vi "SCMain.vi"(0 "once?":bool, 1 "continousSequencer?":bool) -> ()   [LabVIEW 2014]
uses:
  <vilib>/Platform/TimedLoop/XDataNode/timing_clust.ctl
  <vilib>/Platform/TimedLoop/XDataNode/nitl_modes.ctl
  <vilib>/Platform/TimedLoop/XDataNode/wakeup.ctl
  SCGlobVars.vi
  <vilib>/rvi/Emulation/niFpgaSctlEmulationGetInTimedLoop.vi
  <vilib>/rvi/Emulation/niFpgaEmulationReportErrorSimple.vi
  <vilib>/rvi/Emulation/niFpgaGetClockAttributes.vi
  <vilib>/rvi/Emulation/niFpgaCriticalErrorInLSC.vi
  <vilib>/rvi/eio/common/nirviEmuTemplateMethod_errors.vi
  Sequencer/sequencerGlobVars.vi
  <vilib>/Platform/TimedLoop/XDataNode/XDataNode.xnode
  <vilib>/eio/EIONode/EIONode.xnode
  <vilib>/Platform/TimedLoop/XDataNode/XDNodeRunTimeDep.lvlib
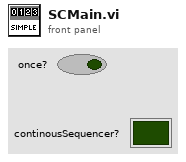
[diagram p1: front panel]
types:
  T1 = typedef "XDNodeRunTimeDep.lvlib/timing_clust.ctl" = cluster{"Expected End [f-1]":u64, "Actual End [f-1]":u64, "Finished Late? [f-1]":bool, "Expected End [i-1]":u64, "Actual End [i-1]":u64, "Finished Late? [i-1]":bool, "Expected Start [i]":u64, "Actual Start [i]":u64, "Expected Start [f]":u64, "Actual Start [f]":u64, "Source Name":string, "Structure Name":string, "Period":i64, "Deadline":i64, "Offset":i64, "Start":i64, "Priority":i32, "Timeout":i32, "Mode":T2, "Wakeup Reason":T3, "Error":errorcluster, "Source Type":string, "Secondary Source Type":string, "Global End Time":u64, "Global Start Time":u64, "Frame Duration":u64, "Iteration Duration":u64, "Assigned CPU":i32, "I/O Scan Engine Mode":u32}
  T2 = typedef "XDNodeRunTimeDep.lvlib/nitl_modes.ctl" = enum32{"No Change", "Process missed periods, maintain original phase", "Discard missed periods, maintain original phase", "Process missed periods, ignore original phase", "Discard missed periods, ignore original phase"}
  T3 = typedef "XDNodeRunTimeDep.lvlib/wakeup.ctl" = enum32{"Normal", "Aborted", "Asynchronous wakeup", "Timing source error", "Timed loop error", "Timeout"}
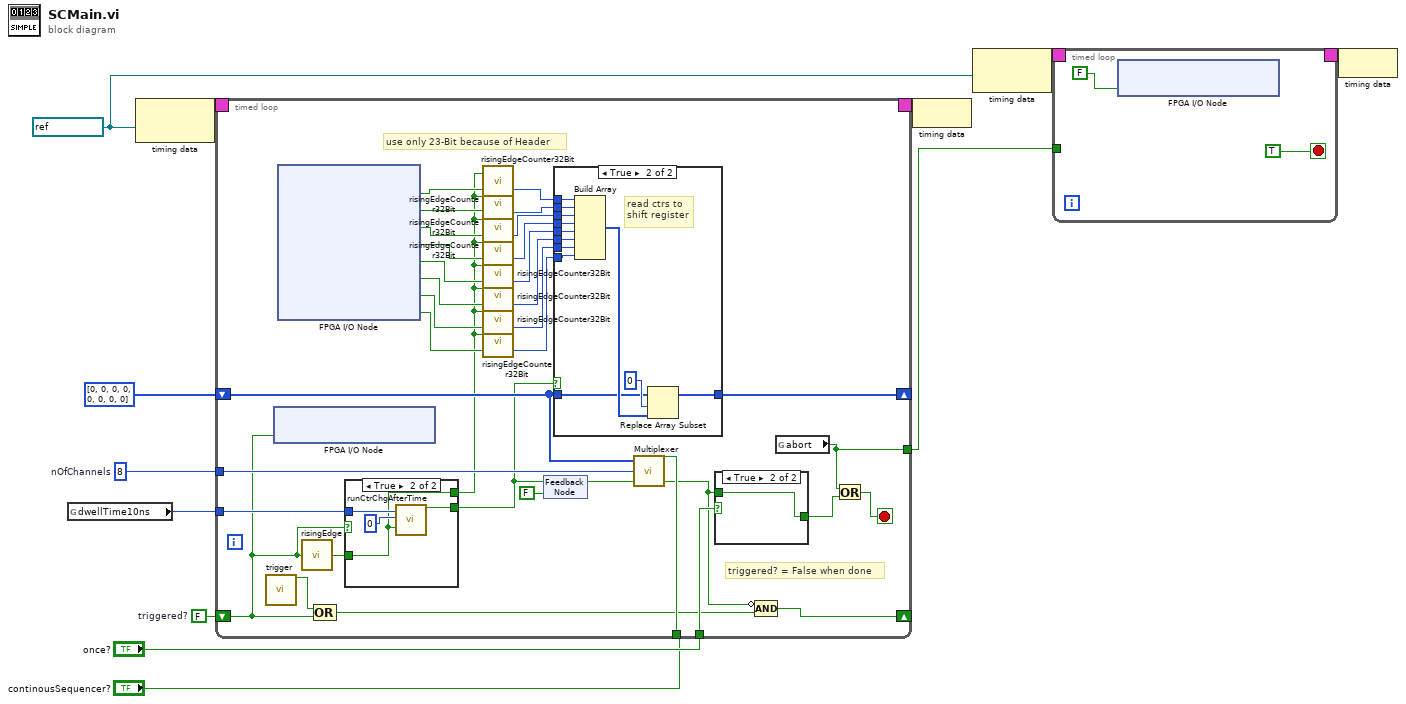
[diagram p0: block diagram]
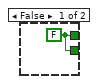
[diagram p2: hidden frame]
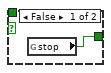
[diagram p3: hidden frame]
diagram:
  w1 = FALSE  # triggered?
  w9 = u8 8  # nOfChannels
  w3 = refnum<k21> "100MHz" ("Source Name")
  n1 = global read "SCGlobVars.vi" "dwellTime10ns"() -> (w5:u32)
  n2 = node-c288(w3) -> (w12:T1)
  n3 = timed-loop {
    timing: w12 -> [_]
    timing-out: [_] -> w11
    shift-right: [w31] -> _
    shift-left: u32[] [0, 0, 0, 0, 0, 0, 0, 0] -> [w28]
    tunnel: w9 -> [w26]
    tunnel: w5 -> [w30]
    tunnel: "once?" -> [w25]
    tunnel: "continousSequencer?" -> [w24]
    tunnel: [w21] -> w2
    shift-right: [w19] -> _
    shift-left: w1 -> [w13]
    stop <- w22 stop-if-true
    # "triggered? = False when done"
    # "use only 23-Bit because of Header"
    n4 = call "trigger.vi"() -> ("triggered"=w20:bool)  [unwired: 19 in]
    n5 = xnode "FPGA I/O Node"("SPScanFlagDio11Con1"=w13) -> ()  [unwired: 1 in, 1 out]
    n6 = xnode "FPGA I/O Node"() -> ("Connector1/DIO16"=w47:bool, "Connector1/DIO17"=w46:bool, "Connector1/DIO18"=w45:bool, "Connector1/DIO19"=w44:bool, "Connector1/DIO20"=w43:bool, "Connector1/DIO21"=w42:bool, "Connector1/DIO22"=w41:bool, "Connector1/DIO23"=w40:bool)  [unwired: 8 in, 8 out]
    n7 = call "risingEdge.vi"("In"=w13) -> ("out"=w14:bool)
    n8 = Compound Arithmetic op=OR(w20, w13) -> (w18:bool)
    n9 = case shown="True" w13 {
      tunnel: w30 -> [_ w52]
      tunnel: [w48 w49] -> w17
      tunnel: [w48 w50] -> w16
      tunnel: w14 -> [_ w49]
      frame False {
        w48 = FALSE ("out")
      }
      frame True {
        n10 = call "runCtrChgAfterTime.vi"("timeDif(ticks)"=w52, "init(ticks)"=u32 0, "forceReset"=w49) -> ("change"=w50:bool)  [unwired: 16 in]
      }
    }
    n11 = call "risingEdgeCounter32Bit.vi"("In"=w47, "Reset"=w17) -> ("32BitCounter"=w39:u32)  [unwired: 1 in]
    n12 = call "risingEdgeCounter32Bit.vi"("In"=w46, "Reset"=w17) -> ("32BitCounter"=w38:u32)  [unwired: 1 in]
    n13 = call "risingEdgeCounter32Bit.vi"("In"=w45, "Reset"=w17) -> ("32BitCounter"=w37:u32)  [unwired: 1 in]
    n14 = call "risingEdgeCounter32Bit.vi"("In"=w44, "Reset"=w17) -> ("32BitCounter"=w36:u32)  [unwired: 1 in]
    n15 = call "risingEdgeCounter32Bit.vi"("In"=w43, "Reset"=w17) -> ("32BitCounter"=w35:u32)  [unwired: 1 in]
    n16 = call "risingEdgeCounter32Bit.vi"("In"=w42, "Reset"=w17) -> ("32BitCounter"=w34:u32)  [unwired: 1 in]
    n17 = call "risingEdgeCounter32Bit.vi"("In"=w41, "Reset"=w17) -> ("32BitCounter"=w33:u32)  [unwired: 1 in]
    n18 = call "risingEdgeCounter32Bit.vi"("In"=w40, "Reset"=w17) -> ("32BitCounter"=w32:u32)  [unwired: 1 in]
    n19 = feedback-in #1(w16) -> ()
    n20 = feedback #1(FALSE ("change")) -> (w27:bool)
    n21 = case shown="True" w16 {
      tunnel: w39 -> [_ w67]
      tunnel: w38 -> [_ w66]
      tunnel: w37 -> [_ w65]
      tunnel: w36 -> [_ w64]
      tunnel: w35 -> [_ w63]
      tunnel: w34 -> [_ w62]
      tunnel: w33 -> [_ w61]
      tunnel: w32 -> [_ w60]
      tunnel: [w55 w57] -> w31
      tunnel: w28 -> [w55 w56]
      frame False {
      }
      frame True {
        # "read ctrs to\nshift register"
        n22 = Build Array(w67, w66, w65, w64, w63, w62, w61, w60) -> (w59:u32[])
        n23 = Replace Array Subset(array=w56, new element=w59, index=0) -> (w57:u32[])
      }
    }
    n24 = call "Multiplexer.vi"("continousSequencer?"=w24, "write"=w27, "nOfChannels"=w26, "Data"=w28) -> ("done"=w15:bool)  [unwired: 1 in]
    n25 = case shown="True" w25 {
      tunnel: w15 -> [_ w54]
      tunnel: [w53 w54] -> w23
      frame False {
        n26 = global read "SCGlobVars.vi" "stop"() -> (w53:bool)
      }
      frame True {
      }
    }
    n27 = Compound Arithmetic op=AND(invert w15, w18) -> (w19:bool)
    n28 = global read "sequencerGlobVars.vi" "abort"() -> (w21:bool)
    n29 = Or(x=w21, y=w23) -> (x .or. y?=w22:bool)
  }
  n30 = node-c288(w11) -> ()
  n31 = node-c288(w3) -> (w8:T1)
  n32 = timed-loop {
    timing: w8 -> [_]
    timing-out: [_] -> w7
    tunnel: w2 -> [_]
    stop <- TRUE stop-if-true
    n33 = xnode "FPGA I/O Node"("SPScanFlagDio11Con1"=FALSE) -> ()  [unwired: 1 in, 1 out]
  }
  n34 = node-c288(w7) -> ()
